vi "Create Message Queue.vi"(8 "error in (no error)":errorcluster, 10 "Max Size (100)":i32=100, 11 "Queue Name":string) -> (0 "error out":errorcluster, 3 "queue out":refnum<queue>)   [LabVIEW 2018, in "Messaging.lvlib"]
uses:
  Messaging.lvlib
  Message Cluster.ctl
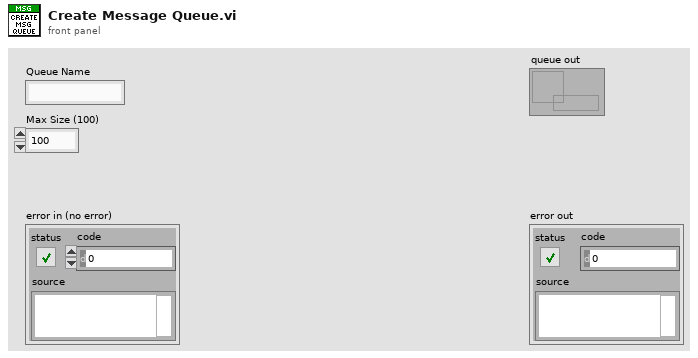
[diagram p1: front panel]
types:
  T1 = typedef "Messaging.lvlib/Message Cluster.ctl" = cluster{"Event":string, "Source":string, "Target":string, "Data":variant}
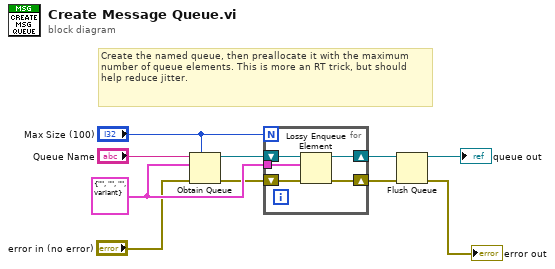
[diagram p0: block diagram]
diagram:
  w9 = T1 {"Event"="", "Source"="", "Target"="", "Data"=variant} ("Message")
  # "Create the named queue, then preallocate it with the maximum number of queue elements. This is more an RT trick, but should help reduce jitter."
  n1 = Obtain Queue(max queue size (-1, unlimited)="Max Size (100)", name (unnamed)="Queue Name", element data type=w9, error in (no error)="error in (no error)") -> (queue out=w7:refnum<queue>, error out=w3:errorcluster)  [unwired: 1 in, 1 out]
  n2 = for {
    N: "Max Size (100)" -> [_]
    shift-right: [w14] -> w10
    shift-left: w7 -> [w15]
    tunnel: w9 -> [w13]
    shift-right: [w11] -> w2
    shift-left: w3 -> [w12]
    n3 = Lossy Enqueue Element(queue=w15, element=w13, error in (no error)=w12) -> (queue out=w14:refnum<queue>, error out=w11:errorcluster)  [unwired: 2 out]
  }
  n4 = Flush Queue(queue=w10, error in (no error)=w2) -> (queue out=→"queue out":refnum<queue>, error out=→"error out":errorcluster)  [unwired: 1 out]
